vi "mass_flow_rate.vi"(2 "Density":dbl[](array[numeric]), 3 "dP H2O":dbl[](array[numeric])) -> (0 "Mass Flow Rate [g/s] Array":dbl[](array[numeric]), 1 "Mass Flow Rate [g/s]":dbl)   [LabVIEW 2015]
uses:
  <vilib>/express/express arith-compare/Formula/XNode/ExpressFormulaBlockNode.xnode
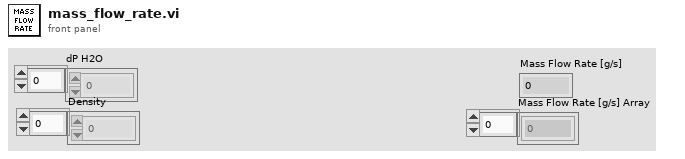
[diagram p1: front panel]
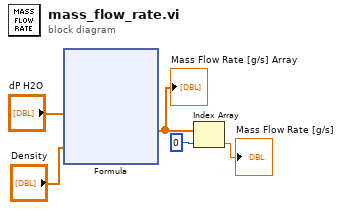
[diagram p0: block diagram]
diagram:
  n1 = xnode "Formula"("rho"="dP H2O", "dP"="Density") -> ("Result"=w1:dbl[])  [unwired: 1 in, 1 out]
  "Mass Flow Rate [g/s] Array" <- w1
  n2 = Index Array(array=w1, index=0) -> (element=→"Mass Flow Rate [g/s]":dbl)
